vi "Saludo.vi"(8 "error in (no error)":errorcluster, 11 "FirstActor in":refnum<class "FirstActor.lvclass">) -> (0 "error out":errorcluster, 3 "FirstActor out":refnum<class "FirstActor.lvclass">)   [LabVIEW 2020, in "FirstActor.lvlib" / "FirstActor.lvclass"]
uses:
  FirstActor.lvclass
  FirstActor.lvclass/FirstActor.ctl
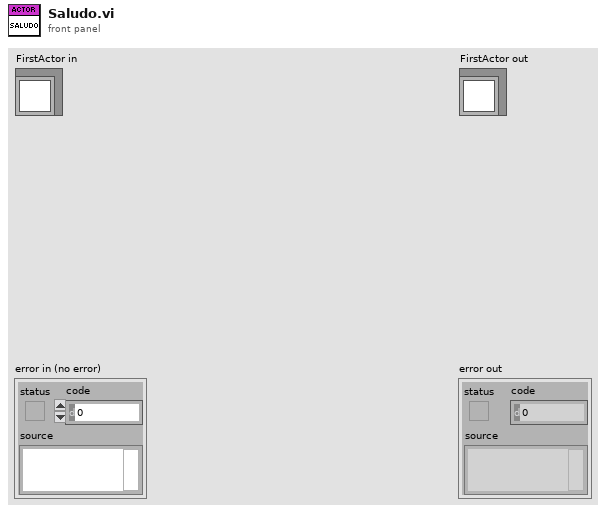
[diagram p1: front panel]
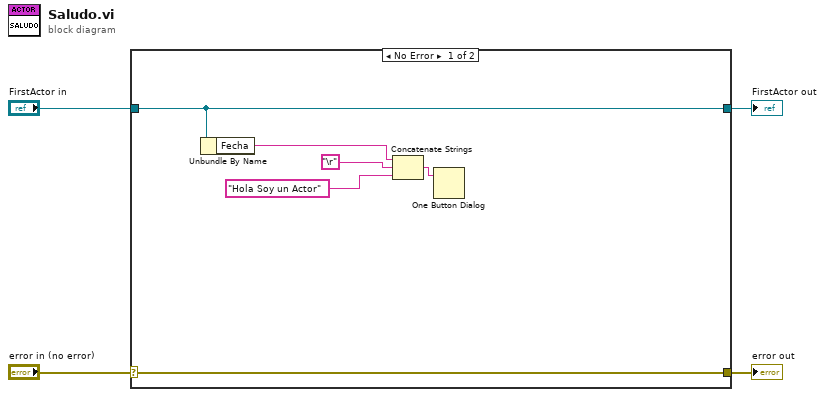
[diagram p0: block diagram]
diagram:
  n1 = case shown="No Error" "error in (no error)" {
    selector: "error in (no error)" -> [w10 w12]
    tunnel: [w10 w12] -> w3
    tunnel: [w8 w11] -> w1
    tunnel: "FirstActor in" -> [w8 w11]
    frame No Error {
      n2 = Unbundle By Name(w8) -> ("Fecha"=w6:string)
      n3 = Concatenate Strings(w6, "\r", "Hola Soy un Actor" ("message")) -> (w7:string)
      n4 = One Button Dialog(message=w7) -> ()  [unwired: 1 in, 1 out]
    }
    frame Error {
    }
  }
  "error out" <- w3
  "FirstActor out" <- w1
